vi "Initialize.vi"(11 "ThisContext":i32) -> (0 "error out":errorcluster, 3 "refnum":T1)   [LabVIEW 2025, in "xTest.lvlib"]
uses:
  xTest.lvlib
  ContextProxy.ctl
  D:/xTestPlatform/xTestPlatform/bin/x86/Debug/net8.0-windows/win-x86/xTestPlatform.Interop.dll
  xTestPlatform/bin/x86/Debug/net8.0-windows/win-x86/xTestPlatform.Interop.dll
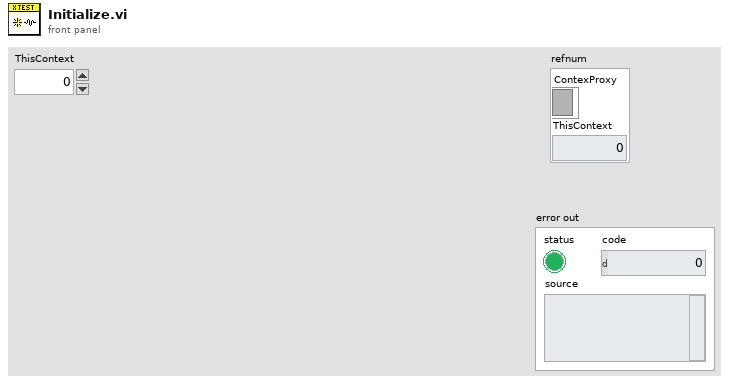
[diagram p1: front panel]
types:
  T1 = typedef "xTest.lvlib/ContextProxy.ctl" = cluster{"ContexProxy":refnum<k39>, "ThisContext":i32}
  T2 = cluster{"new reference":refnum<k39>, "ThisContext":i32}
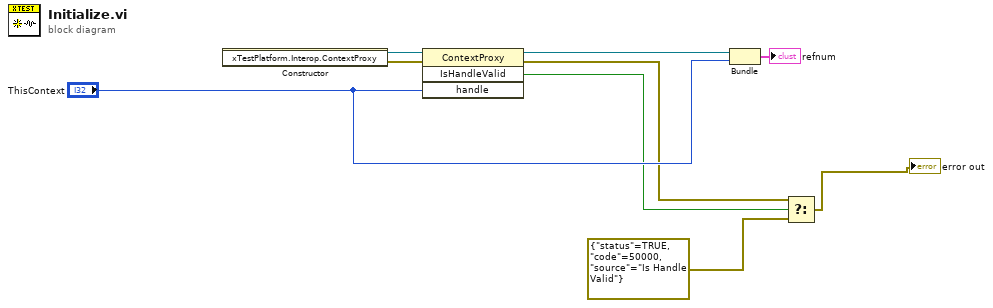
[diagram p0: block diagram]
diagram:
  n1 = constructor class="ContextProxy"() -> (reference out=w9:refnum<k39>, error out=w8:errorcluster)  [unwired: 3 in, 1 out]
  n2 = invoke class="ContextProxy" method="IsHandleValid"(reference=w9, error in=w8, "handle"="ThisContext") -> (reference out=w7:refnum<k39>, error out=w3:errorcluster, "IsHandleValid"=w4:bool)  [unwired: 1 in, 1 out]
  n3 = Bundle("new reference"=w7, "ThisContext"="ThisContext") -> (→"refnum":T2)  [unwired: 1 in]
  n4 = Select(t=w3, s=w4, f=errorcluster {"status"=TRUE, "code"=50000, "source"="Is Handle Valid"}) -> (s? t:f=→"error out":errorcluster)
